vi "Custom_XOR.vi"(9 "INPUT B":bool, 11 "INPUT A":bool) -> (3 "Boolean 3":bool)   [LabVIEW 2026]
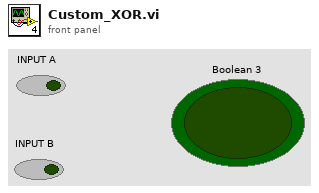
[diagram p1: front panel]
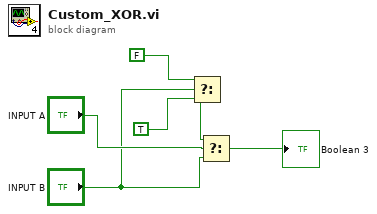
[diagram p0: block diagram]
diagram:
  n1 = Select(t=FALSE, s="INPUT B", f=TRUE) -> (s? t:f=w1:bool)
  n2 = Select(t=w1, s="INPUT A", f="INPUT B") -> (s? t:f=→"Boolean 3":bool)
